vi "公式.vi"(7 "功能":enum16{"读取", "写入"}(ring), 8 "error in (no error)":errorcluster caption="错误输入（无错误）", 10 "公式写入":cluster{"X^2":dbl, "X":dbl, "b":dbl}, 11 "MB session in":refnum<class "MB_Master.lvclass">) -> (0 "error out":errorcluster caption="错误输出", 2 "公式读取":cluster{"X^2":dbl, "X":dbl, "b":dbl}, 3 "MB session out":refnum<class "MB_Master.lvclass">)   [LabVIEW 2016, in "斯坦道总磷.lvlib"]
uses:
  <vilib>/Plasmionique/MB Master/MB_Master/MB_Master.lvclass
  <vilib>/Plasmionique/MB Master/MB Master.lvlib
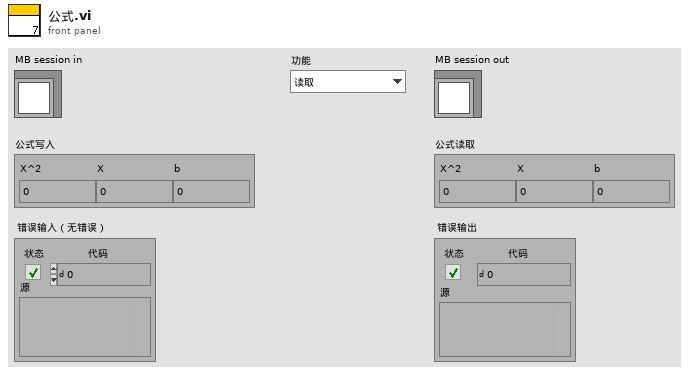
[diagram p1: front panel]
types:
  T1 = cluster{"FLOAT[0]":sgl, "FLOAT[1]":sgl, "FLOAT[2]":sgl}
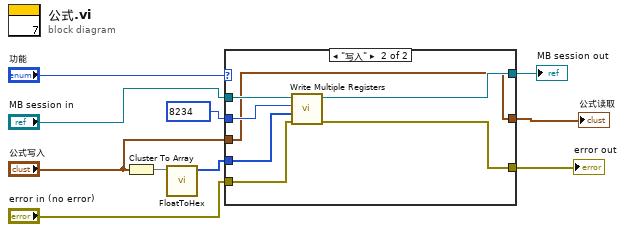
[diagram p0: block diagram]
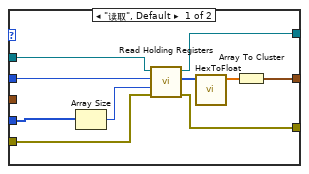
[diagram p2: hidden frame]
diagram:
  n1 = Cluster To Array(cluster="公式写入") -> (array=w6:dbl[])
  n2 = call "FloatToHex.vi"("浮点数"=w6) -> ("DCBA整形输出"=w5:u16[])  [unwired: 10 in]
  n3 = case shown="\"写入\"" "功能" {
    tunnel: "error in (no error)" -> [w17 w27]
    tunnel: [w18 w26] -> w9
    tunnel: [w19 w25] -> w8
    tunnel: u16 8234 ("starting address") -> [w16 w24]
    tunnel: w5 -> [w15 w23]
    tunnel: "MB session in" -> [w20 w22]
    tunnel: [w11 w21] -> w1
    tunnel: "公式写入" -> [_ w21]
    frame "读取", Default {
      n4 = Array Size(array=w15) -> (size(s)=w14:i32)
      n5 = call <vilib>:"Read Holding Registers.vi"("error in (no error)"=w17, "quantity"=w14, "starting address"=w16, "MB session in"=w20) -> ("error out"=w18:errorcluster, "Registers"=w12:u16[], "MB session out"=w19:refnum<class "MB_Master.lvclass">)  [unwired: 5 in]
      n6 = call "HexToFloat.vi"("数组"=w12) -> ("FLOAT"=w13:sgl[])  [unwired: 10 in]
      n7 = Array To Cluster(array=w13) -> (cluster=w11:T1)
    }
    frame "写入" {
      n8 = call <vilib>:"Write Multiple Registers.vi"("error in (no error)"=w27, "values"=w23, "starting address"=w24, "MB session in"=w22) -> ("error out"=w26:errorcluster, "MB session out"=w25:refnum<class "MB_Master.lvclass">)  [unwired: 6 in]
    }
  }
  "error out" <- w9
  "MB session out" <- w8
  "公式读取" <- w1
